vi "FileExplorer.vi"(0 "FolderPath":path, 1 "Copy Button":bool, 2 "Expand/Collapse":bool, 5 "Tree":string[](tree), 7 "SearchBar":string, 11 "error in (no error)":errorcluster) -> (4 "Report":string, 15 "error out":errorcluster)   [LabVIEW 2021]
doc: "This Vi acts as a file explorer. It populates the subfolders and files present in the selected folder path in tree along with the data of Last Modified,Type and Size of files."
uses:
  Controls/Operations.ctl
  Controls/Data Cluster.ctl
  Controls/State.ctl
panel:
  # "Instructions:\n\n-> Select the folder path to populate the subfolders and files present in tree.\n-> A report is generated for the folders whose checkbox is selected in tree.\n-> Press Collapse All button to collapse all nodes in tree and Expand All to expand\n      all nodes in tree.\n->  Enter a folder name in search bar and click enter to expand the nodes of searched folder.\n-> Click column headers such as Last Modified to sort the column itemns in ascending \n      and descending order.\n-> Select file to copy and click Copy button which opens a dialog box to choose the\n      folder path where the files are copied."
  # "Instructions:\n\n-> Select the Folder Path to populate the subfolders and files present in it in tree.\n->  Can select multiple files of same folder and press Copy button to copy those files.\n->  Clicking a Copy button opens a dialog box to choose the destination folder path \n       where the files are copied.\n->  A report is generated for the folders whose checkbox is selected in tree.\n->  Press Collapse All button to collapse all nodes in tree and Expand all to expand \n       all nodes in tree.\n->   Enter a folder name in SearchBar and press Search to search for a particular folder\n       in tree.\n->   Press column headers such as Last Modified to sort the column items in ascending \n        or descending order."
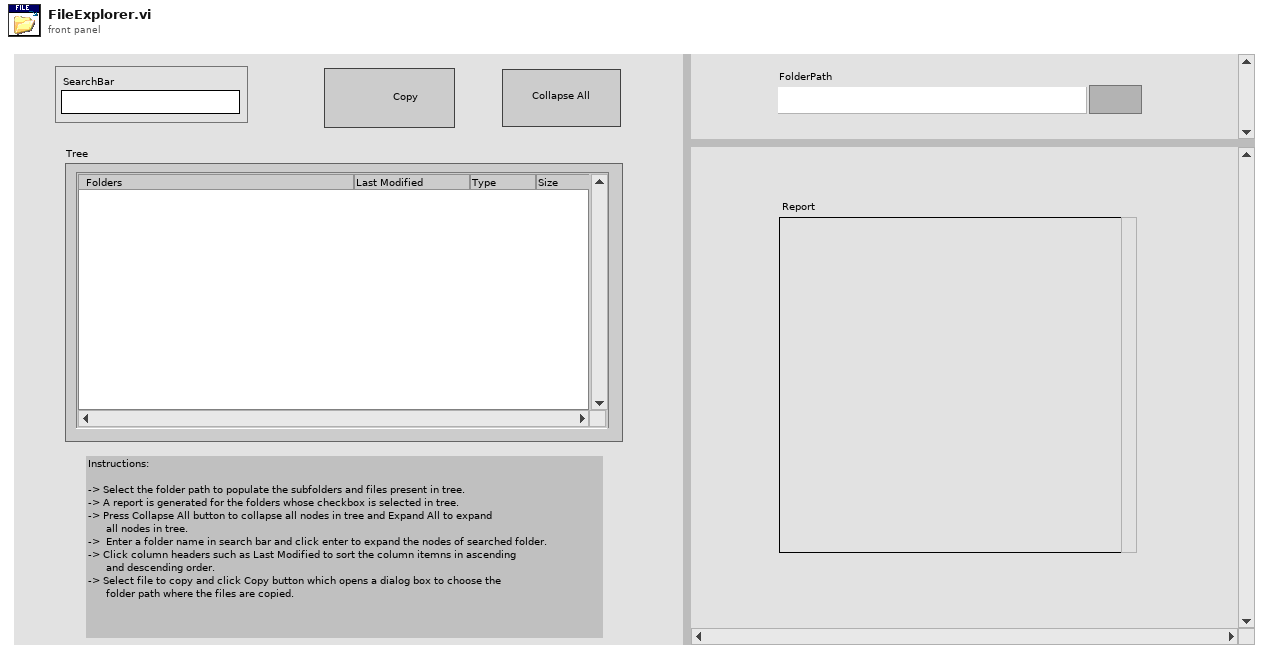
[diagram p1: front panel]
types:
  T1 = typedef "State.ctl" = cluster{"State":string, "Data":variant}
  T2 = typedef "Data Cluster.ctl" = cluster{"Stop user event":refnum<user-event>, "FolderPath":path, "FolderName":string, "FolderPathArray":path[], "FilePathArray":path[], "Index":i32, "No.of Folders":i32, "SelectedTags":string[], "SelectedFilePaths":path[], "SearchTag":string, "Column":i32, "Toggle":bool, "FolderTag":string, "ActiveTag":string, "ListBox":i32, "Report":string, "ValidPath":path, "NewSelectedPath":path}
  T3 = typedef "Operations.ctl" = enum16{"Create", "Enqueue", "Enqueue N", "Enstack", "Dequeue", "Flush", "Release"}
  T4 = typedef "LVPoint32TypeDef.ctl" = cluster{"Horizontal":i32, "Vertical":i32}
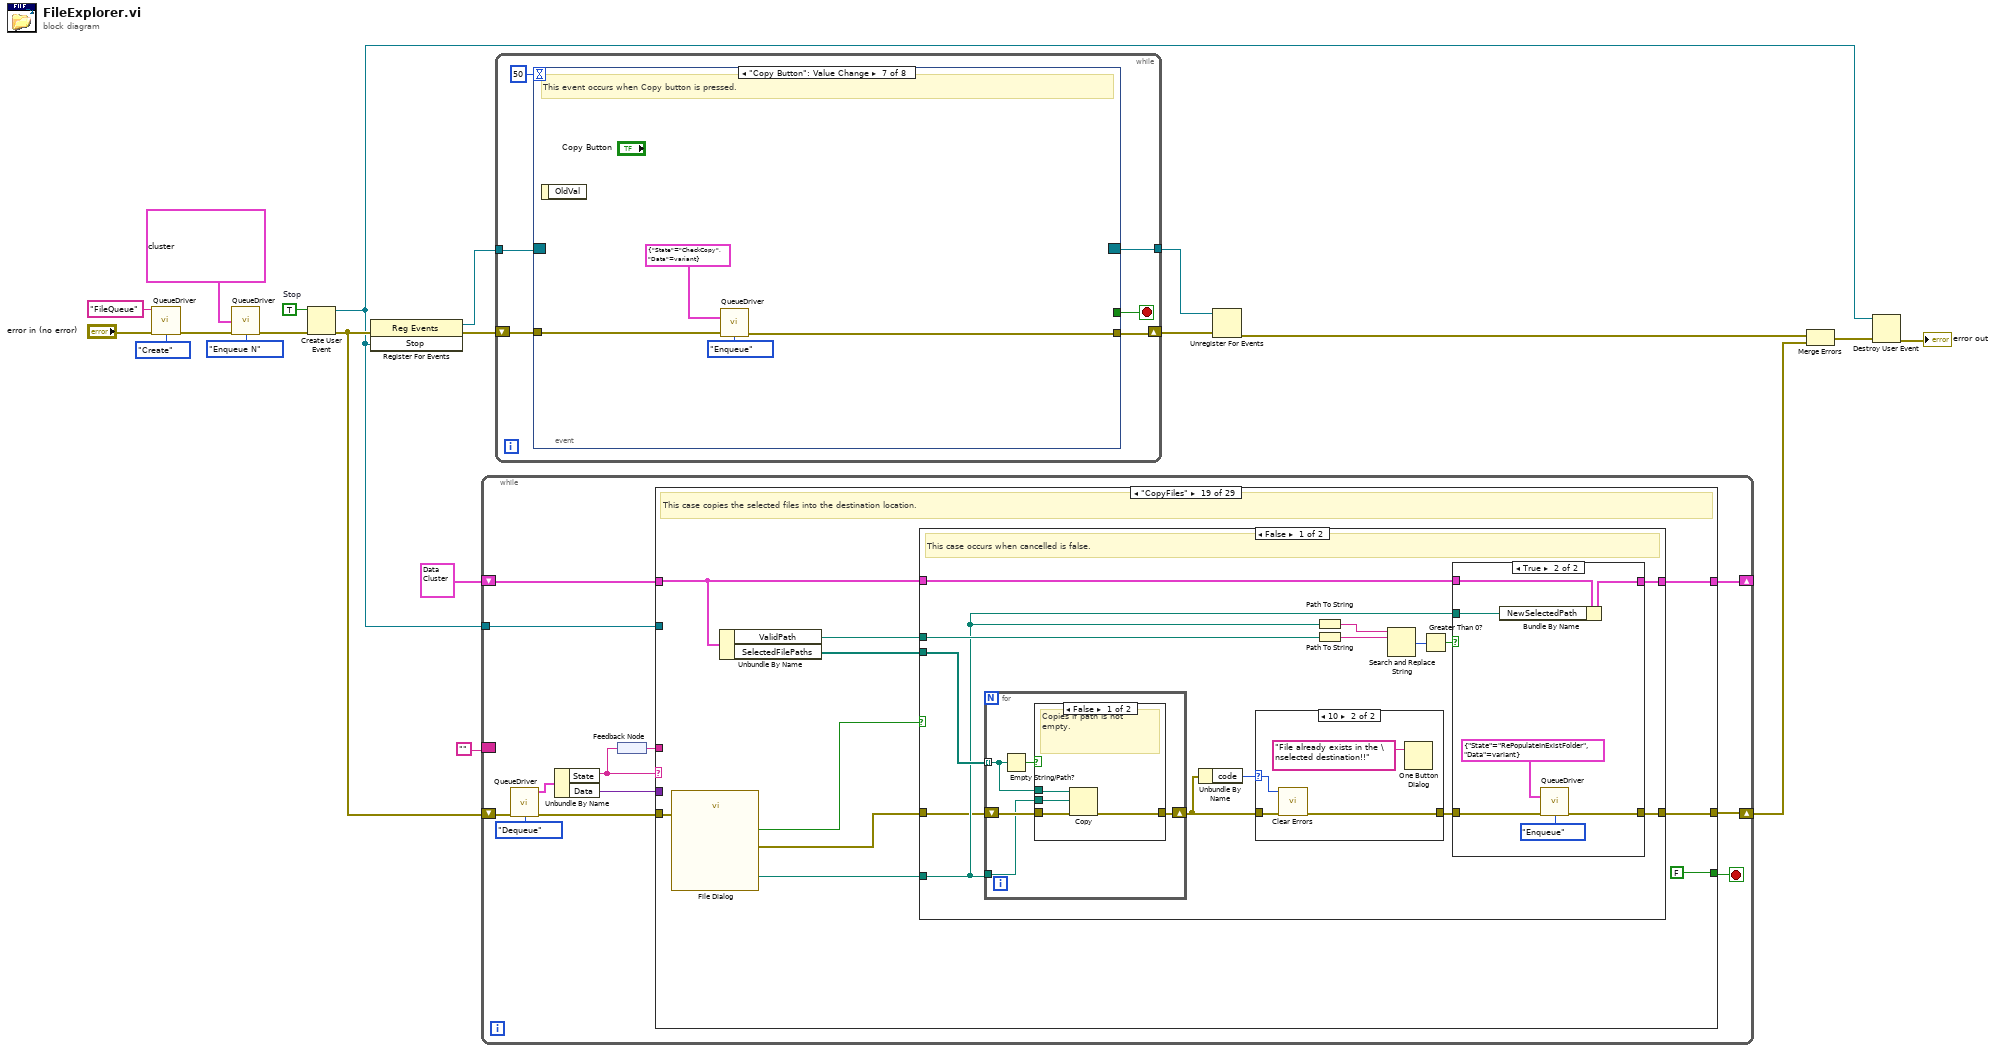
[diagram p0: block diagram]
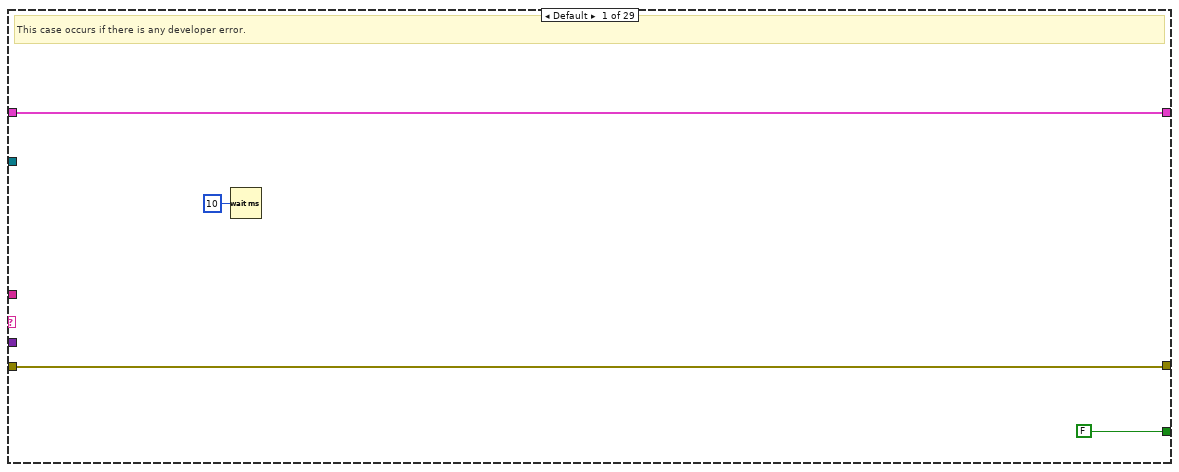
[diagram p2: hidden frame]
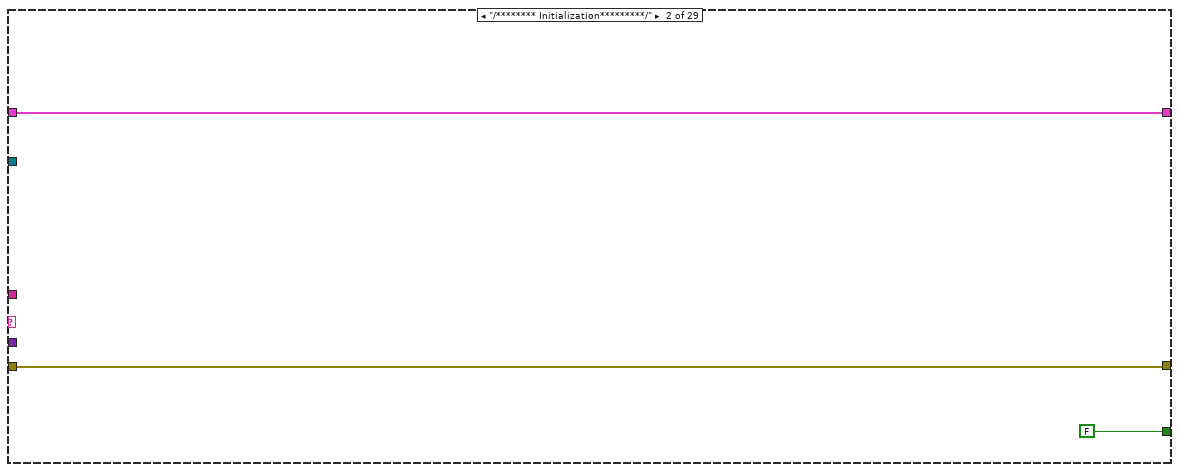
[diagram p3: hidden frame]
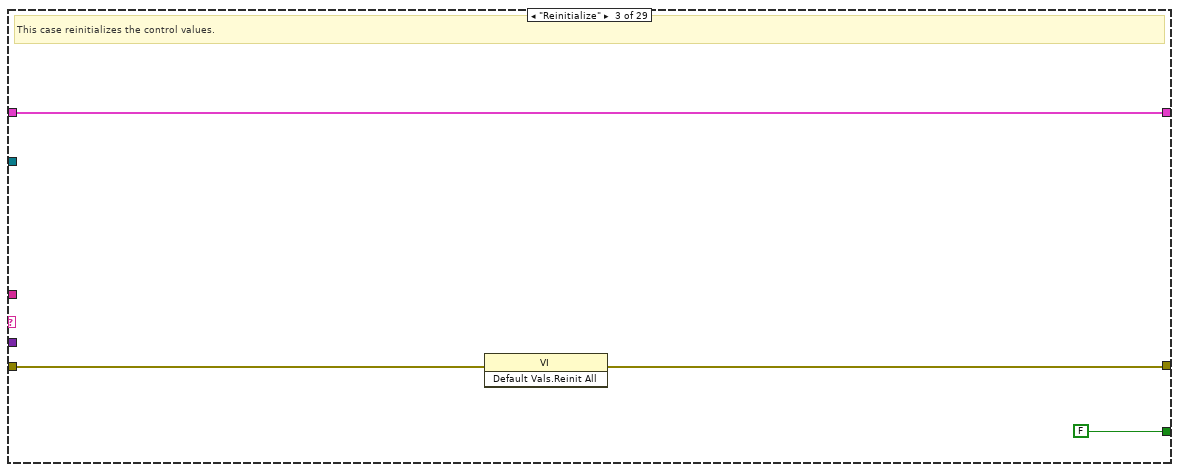
[diagram p4: hidden frame]
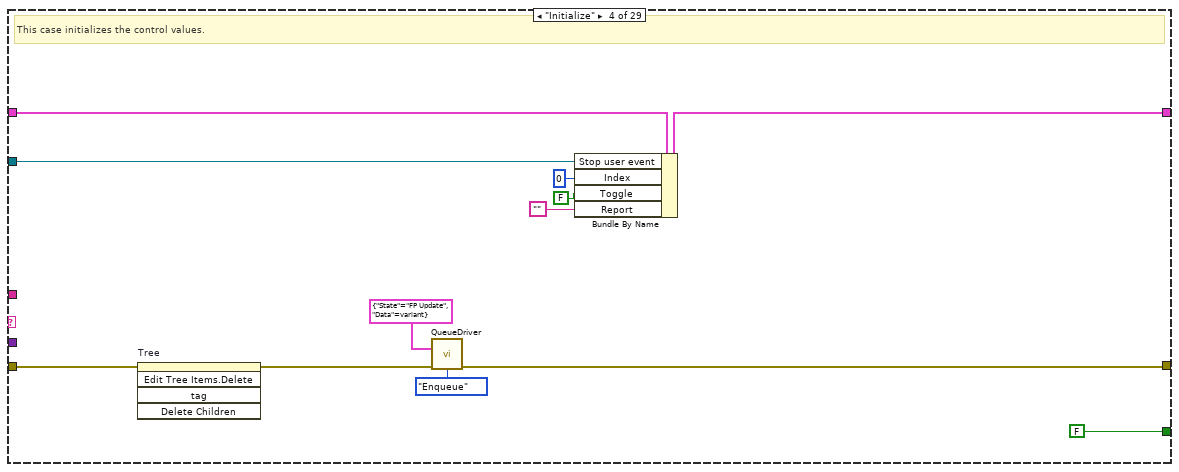
[diagram p5: hidden frame]
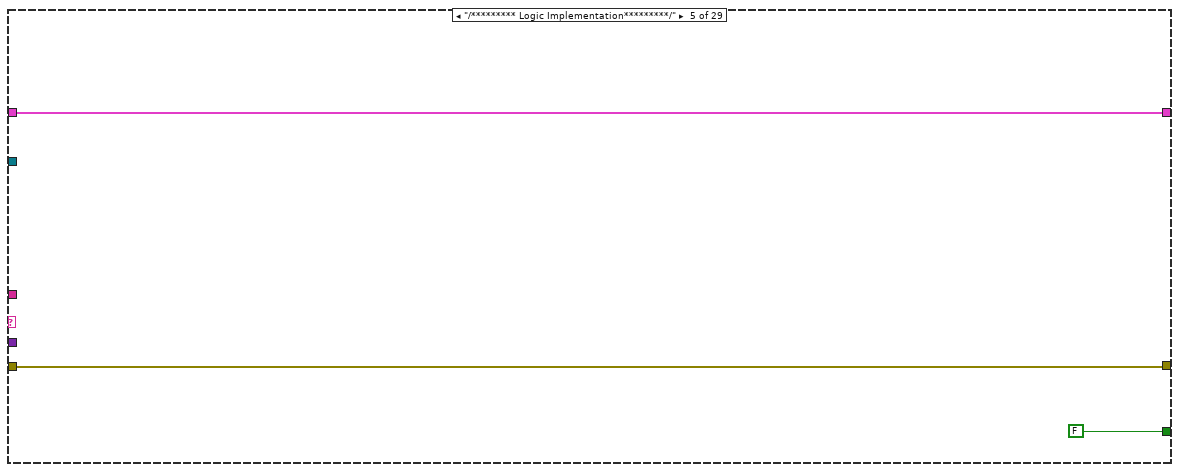
[diagram p6: hidden frame]
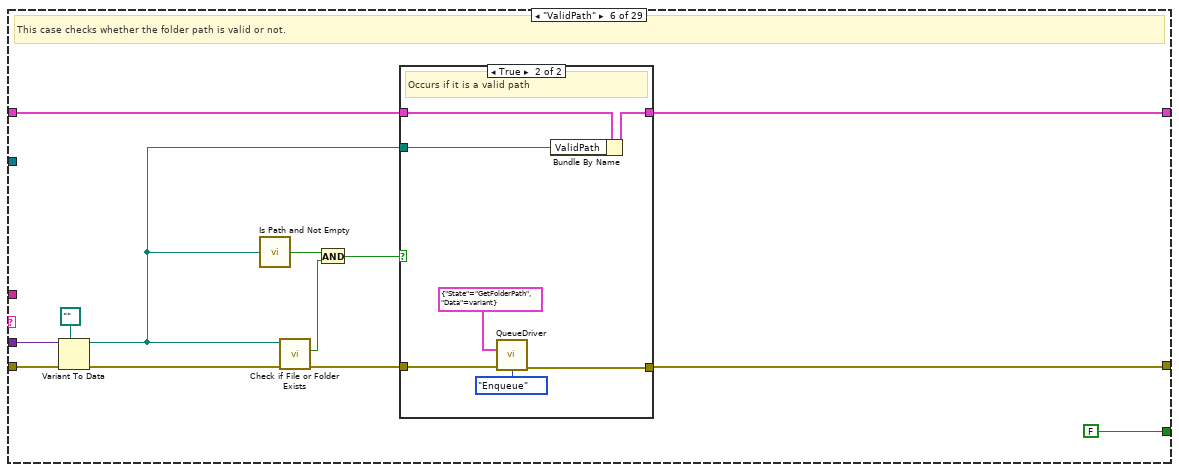
[diagram p7: hidden frame]
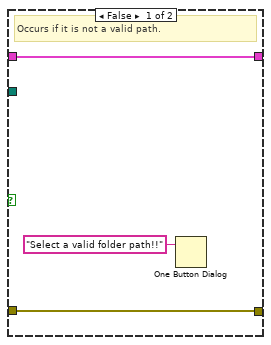
[diagram p8: hidden frame]
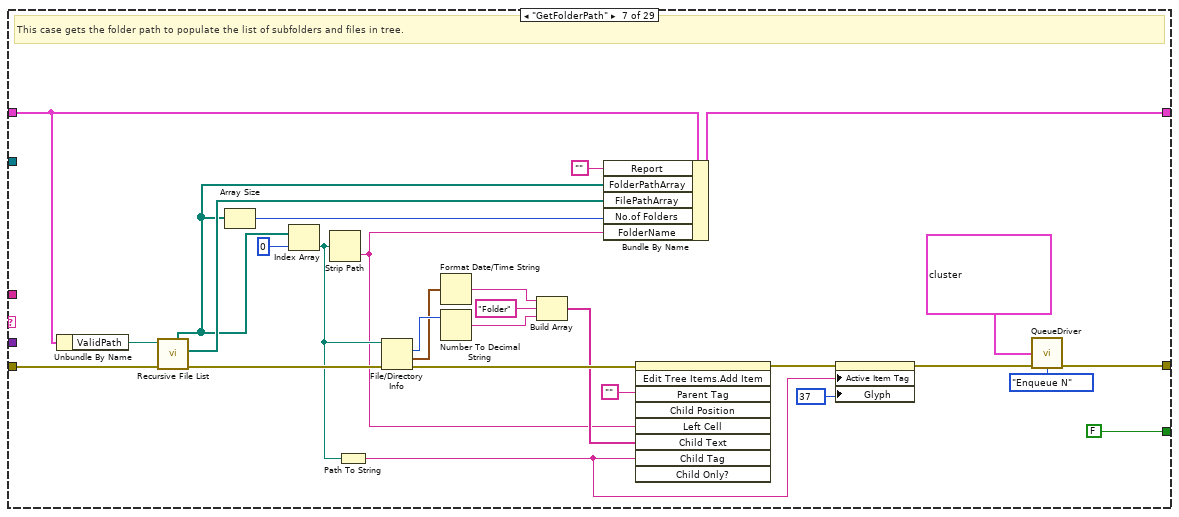
[diagram p9: hidden frame]
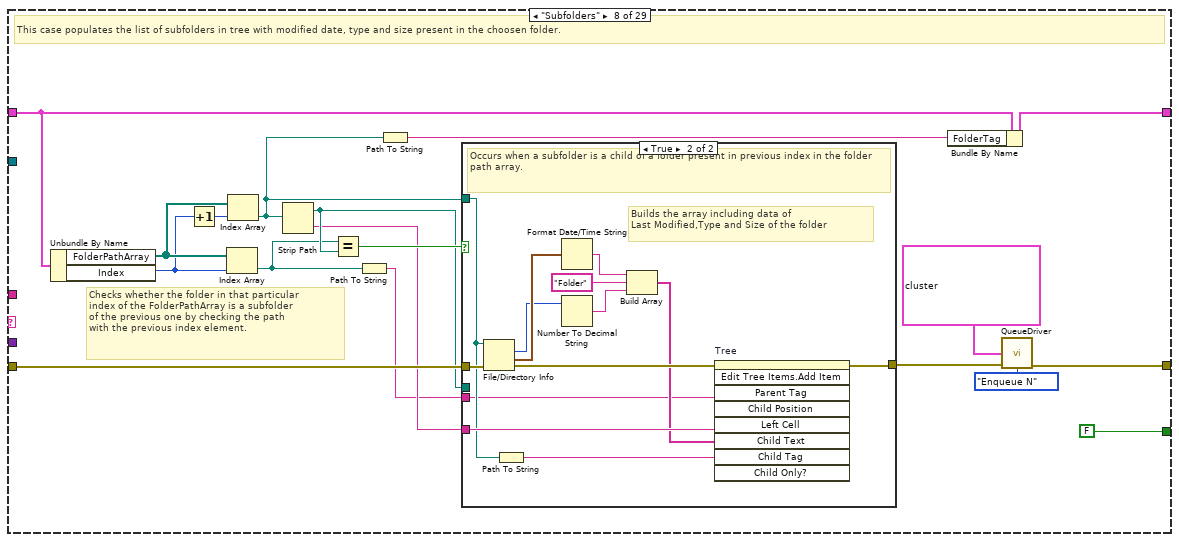
[diagram p10: hidden frame]
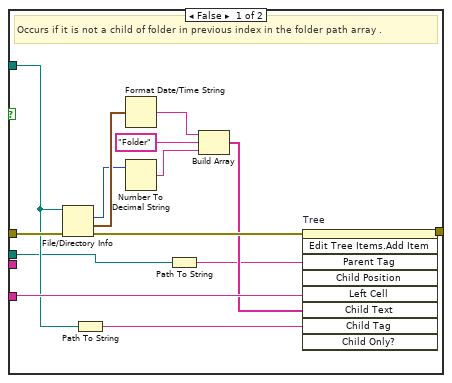
[diagram p11: hidden frame]
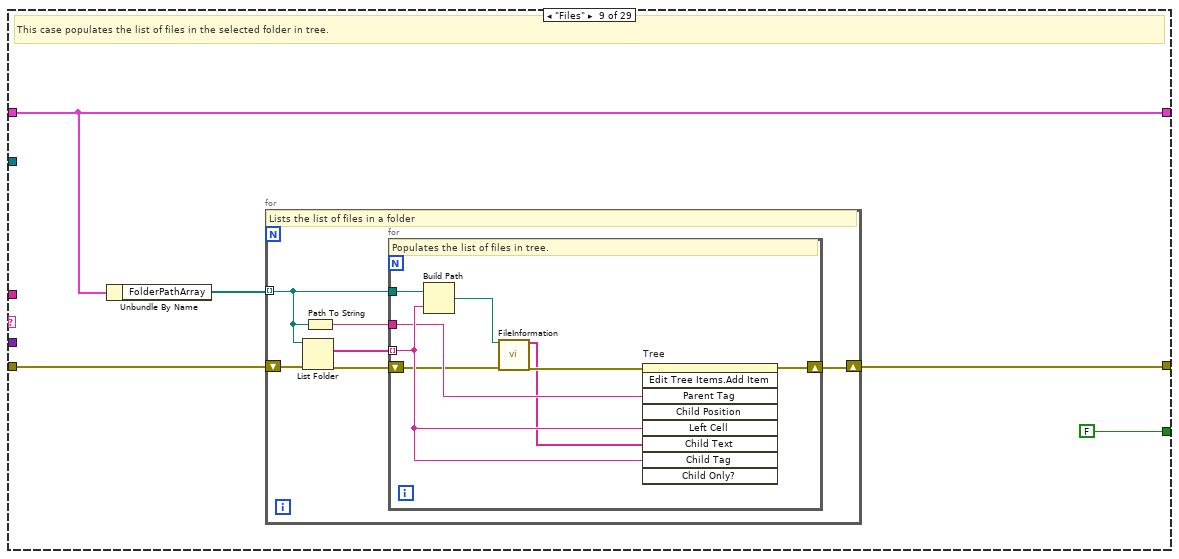
[diagram p12: hidden frame]
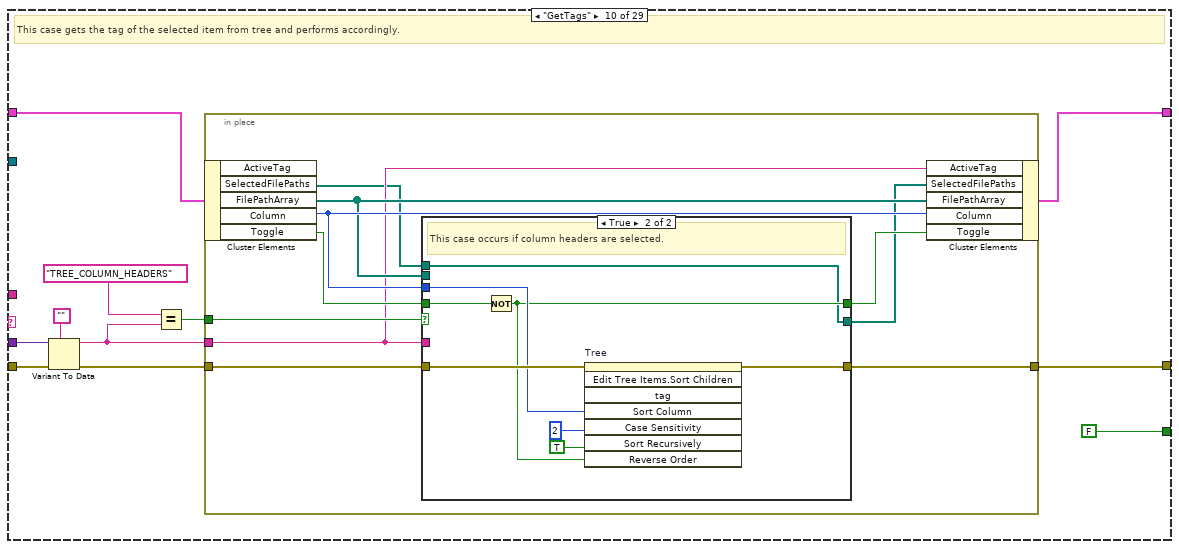
[diagram p13: hidden frame]
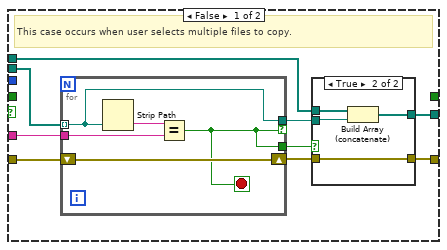
[diagram p14: hidden frame]
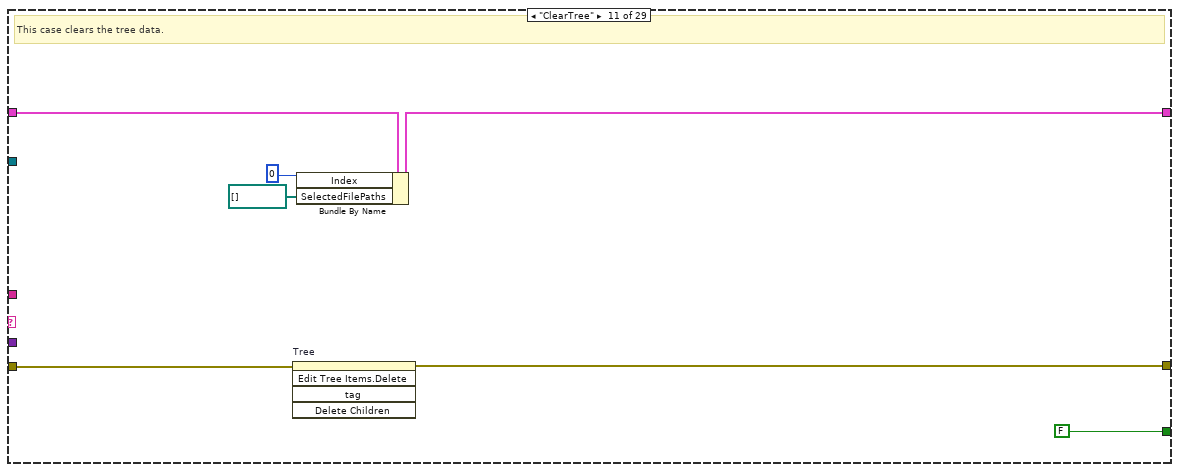
[diagram p16: hidden frame]
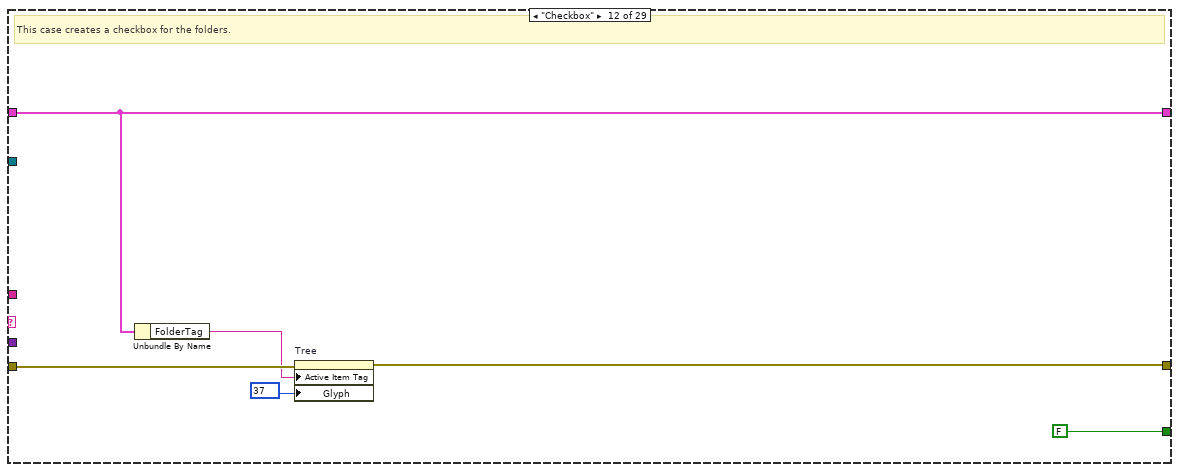
[diagram p17: hidden frame]
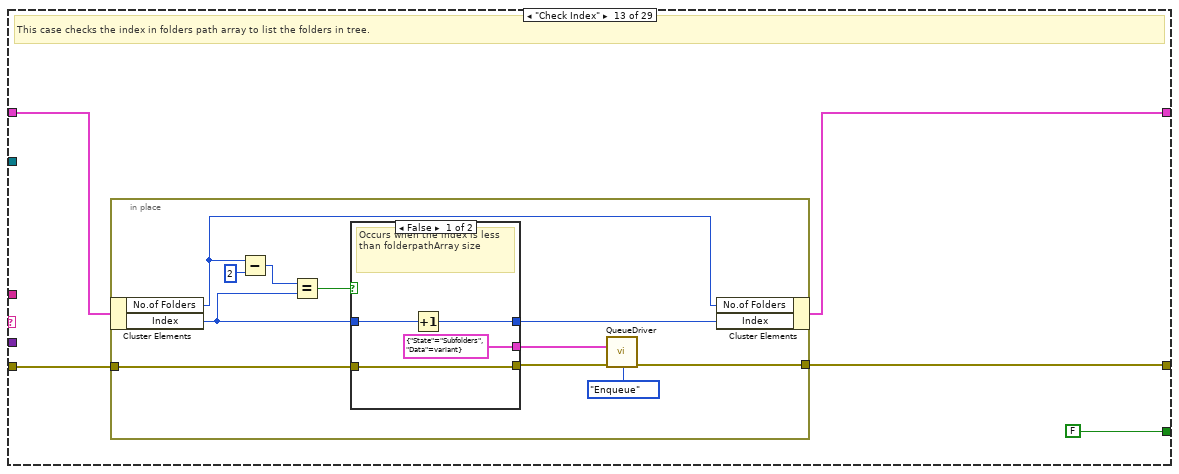
[diagram p18: hidden frame]
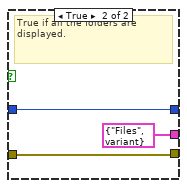
[diagram p19: hidden frame]
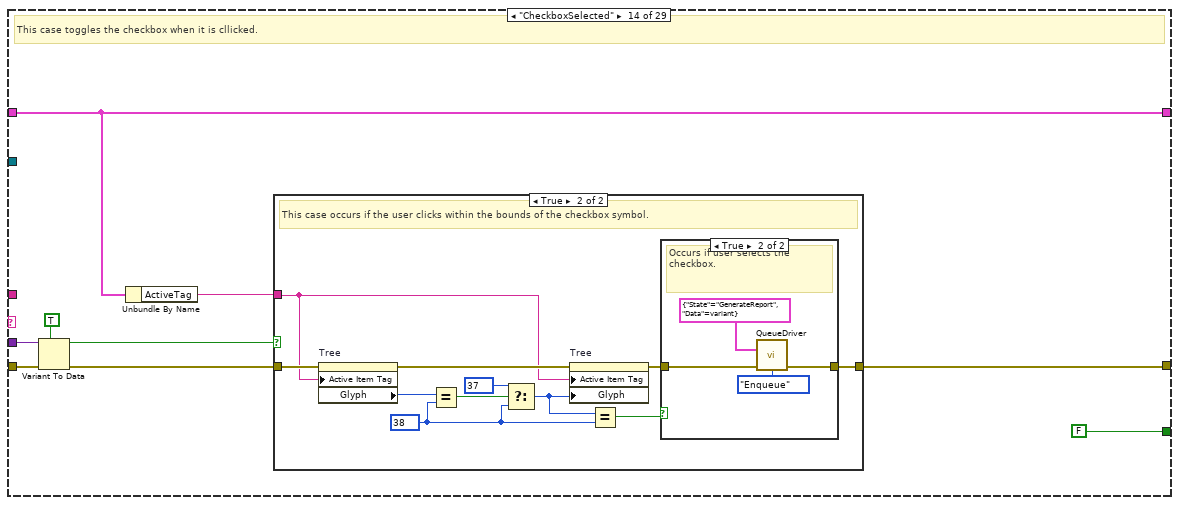
[diagram p20: hidden frame]
diagram:
  w20 = TRUE  # Stop
  n1 = call "QueueDriver.vi"("Queue Name"="FileQueue", "error in (no error)"="error in (no error)", "Operations"=Operations."Create") -> ("error out"=w15:errorcluster)  [unwired: 11 in, 1 out]
  n2 = call "QueueDriver.vi"("State[]"=T1[] [{"State"="Reinitialize", "Data"=variant}, {"State"="Initialize", "Data"=variant}], "error in (no error)"=w15, "Operations"=Operations."Enqueue N") -> ("error out"=w14:errorcluster)  [unwired: 11 in, 1 out]
  n3 = Create User Event(user event datatype=w20, error in=w14) -> (user event=w4:refnum<user-event>, error out=w17:errorcluster)
  n4 = register-events(error in=w17, w4) -> (reference out=w18:refnum<event-registration>, error out=w19:errorcluster)  [unwired: 1 in]
  n5 = while {
    shift-right: [w29] -> w6
    shift-left: w17 -> [w27]
    border: "" ("Empty String Constant") -> [_]
    tunnel: w4 -> [w23]
    shift-right: [w21] -> _
    shift-left: T2 {"Stop user event"=refnum, "FolderPath"=path "", "FolderName"="", "FolderPathArray"=[], "FilePathArray"=[], "Index"=0, "No.of Folders"=0, "SelectedTags"=[], "SelectedFilePaths"=[], "SearchTag"="", "Column"=0, "Toggle"=FALSE, "FolderTag"="", "ActiveTag"="", "ListBox"=0, "Report"="", "ValidPath"=path "", "NewSelectedPath"=path ""} -> [w22]
    stop <- w28 stop-if-true
    n6 = call "QueueDriver.vi"("error in (no error)"=w27, "Operations"=Operations."Dequeue") -> ("Dequeued Element"=w25:T1, "error out"=w26:errorcluster)  [unwired: 12 in]
    n7 = Unbundle By Name(w25) -> ("State"=w32:string, "Data"=w30:variant)
    n8 = feedback-in #1(w32) -> ()
    n9 = feedback #1() -> (w31:string)
    n10 = case shown="\"CopyFiles\"" w32 {
      tunnel: w26 -> [w36 w39 w43 w52 w58 w71 w109 w124 w158 w184 w228 w234 w240 w267 w307 w323 w332 w356 w373 w428 w466 w501 w509 w512 w516 w519 w525 w545 w550]
      tunnel: w31 -> [_ _ _ _ _ _ _ _ _ _ _ _ _ _ _ _ _ _ _ _ _ _ _ _ _ _ w524 _ _]
      tunnel: w30 -> [_ _ _ _ _ w70 _ _ _ w183 _ _ _ w266 _ w322 _ _ _ _ _ w499 w507 _ _ _ _ _ _]
      tunnel: [w36 w39 w41 w46 w58 w68 w105 w120 w156 w181 w229 w233 w239 w260 w288 w317 w324 w355 w370 w423 w464 w496 w508 w512 w516 w519 w523 w545 w549] -> w29
      tunnel: [FALSE FALSE FALSE FALSE FALSE FALSE FALSE FALSE FALSE FALSE FALSE FALSE FALSE FALSE FALSE FALSE FALSE FALSE FALSE FALSE FALSE FALSE FALSE FALSE FALSE FALSE FALSE FALSE TRUE] -> w28
      tunnel: w23 -> [_ _ _ w54 _ _ _ _ _ _ _ _ _ _ _ _ _ _ _ _ _ _ _ _ _ _ _ _ _]
      tunnel: w22 -> [w35 w38 w42 w55 w57 w66 w83 w117 w159 w176 w227 w235 w237 w264 w292 w320 w335 w358 w369 w420 w460 w500 w505 w511 w515 w518 w522 w544 w546]
      tunnel: [w35 w38 w42 w53 w57 w65 w108 w116 w159 w175 w226 w235 w236 w264 w291 w319 w335 w358 w368 w419 w459 w500 w503 w511 w515 w518 w522 w544 w546] -> w21
      frame Default {
        # "This case occurs if there is any developer error."
        n11 = Wait (ms)(milliseconds to wait=u32 10) -> ()  [unwired: 1 out]
      }
      frame "/******** Initialization*********/" {
      }
      frame "Reinitialize" {
        # "This case reinitializes the control values."
        n12 = invoke on="Invoke Node" class="VI" method="Default Vals.Reinit All"(error in=w43) -> (error out=w41:errorcluster)  [unwired: 2 in, 2 out]
      }
      frame "Initialize" {
        # "This case initializes the control values."
        n13 = invoke on="Tree" class="Tree (strict)" method="Edit Tree Items.Delete"(error in=w52) -> (error out=w49:errorcluster)  [unwired: 4 in, 4 out]
        n14 = call "QueueDriver.vi"("State"=T1 {"State"="FP Update", "Data"=variant}, "error in (no error)"=w49, "Operations"=Operations."Enqueue") -> ("error out"=w46:errorcluster)  [unwired: 11 in, 1 out]
        n15 = Bundle By Name(cluster=w55, "Stop user event"=w54, "Index"=0, "Toggle"=FALSE, "Report"="" ("Empty String Constant")) -> (w53:T2)
      }
      frame "/********* Logic Implementation*********/" {
      }
      frame "ValidPath" {
        # "This case checks whether the folder path is valid or not."
        n16 = Variant To Data(error in=w71, type=path "", Variant=w70) -> (data=w61:path, error out=w64:errorcluster)
        n17 = call <vilib>:"Is Path and Not Empty.vi"("path"=w61) -> ("Is Path and Not Empty?"=w60:bool)  [unwired: 4 in]
        n18 = call <vilib>:"Check if File or Folder Exists.vi"("error in (no error)"=w64, "path"=w61) -> ("error out"=w63:errorcluster, "file or folder exists?"=w62:bool)  [unwired: 7 in, 1 out]
        n19 = And(x=w60, y=w62) -> (x .and. y?=w59:bool)
        n20 = case shown="True" w59 {
          tunnel: w63 -> [w74 w81]
          tunnel: [w74 w80] -> w68
          tunnel: w66 -> [w72 w77]
          tunnel: w61 -> [_ w76]
          tunnel: [w72 w75] -> w65
          frame False {
            # "Occurs if it is not a valid path."
            n21 = One Button Dialog(message="Select a valid folder path!!") -> ()  [unwired: 1 in, 1 out]
          }
          frame True {
            # "Occurs if it is a valid path"
            n22 = call "QueueDriver.vi"("State"=T1 {"State"="GetFolderPath", "Data"=variant}, "error in (no error)"=w81, "Operations"=Operations."Enqueue") -> ("error out"=w80:errorcluster)  [unwired: 11 in, 1 out]
            n23 = Bundle By Name(cluster=w77, "ValidPath"=w76) -> (w75:T2)
          }
        }
      }
      frame "GetFolderPath" {
        # "This case gets the folder path to populate the list of subfolders and files in tree."
        n24 = Unbundle By Name(w83) -> ("ValidPath"=w82:path)
        n25 = call <vilib>:"Recursive File List.vi"("error in (no error)"=w109, "Folder Path"=w82) -> ("error out"=w98:errorcluster, "All Files in Dir"=w107:path[], "All Folders"=w103:path[])  [unwired: 5 in, 2 out]
        n26 = Array Size(array=w103) -> (size(s)=w102:i32)
        n27 = Index Array(array=w103, index=0) -> (element=w86:path)
        n28 = Strip Path(path=w86) -> (name=w85:string)  [unwired: 1 out]
        n29 = Path To String(path=w86) -> (string=w84:string)
        n30 = File/Directory Info(path=w86, error in=w98) -> (size=w99:i64, last mod=w96:timestamp, error out=w97:errorcluster)  [unwired: 4 out]
        n31 = Format Date/Time String(seconds (now)=w96) -> (date/time string=w95:string)  [unwired: 2 in]
        n32 = Number To Decimal String(number=w99) -> (decimal integer string=w100:string)  [unwired: 1 in]
        n33 = Build Array(w95, "Folder" ("element"), w100) -> (w94:string[])
        n34 = Bundle By Name(cluster=w83, "Report"="" ("Empty String Constant"), "FolderPathArray"=w103, "FilePathArray"=w107, "No.of Folders"=w102, "FolderName"=w85) -> (w108:T2)
        n35 = invoke on="Tree" class="Tree (strict)" method="Edit Tree Items.Add Item"(error in=w97, "Parent Tag"="" ("Empty String Constant"), "Left Cell"=w85, "Child Text"=w94, "Child Tag"=w84) -> (error out=w93:errorcluster)  [unwired: 4 in, 8 out]
        n36 = property on="Tree" class="Tree (strict)"(error in=w93, "Active Item Tag"=w84, "Glyph"=37) -> (error out=w92:errorcluster)  [unwired: 1 in, 1 out]
        n37 = call "QueueDriver.vi"("State[]"=T1[] [{"State"="FP Update", "Data"=variant}, {"State"="Subfolders", "Data"=variant}], "error in (no error)"=w92, "Operations"=Operations."Enqueue N") -> ("error out"=w105:errorcluster)  [unwired: 11 in, 1 out]
      }
      frame "Subfolders" {
        # "Checks whether the folder in that particular\nindex of the FolderPathArray is a subfolder \nof the previous one by checking the path\nwith the previous index element."
        # "This case populates the list of subfolders in tree with modified date, type and size present in the choosen folder."
        n38 = Unbundle By Name(w117) -> ("FolderPathArray"=w127:path[], "Index"=w126:i32)
        n39 = Increment(x=w126) -> (x+1=w125:i32)
        n40 = Index Array(array=w127, index=w126) -> (element=w111:path)
        n41 = Index Array(array=w127, index=w125) -> (element=w113:path)
        n42 = Strip Path(path=w113) -> (stripped path=w122:path, name=w115:string)
        n43 = Equal?(x=w111, y=w122) -> (x = y?=w123:bool)
        n44 = Path To String(path=w111) -> (string=w110:string)
        n45 = Path To String(path=w113) -> (string=w112:string)
        n46 = case shown="True" w123 {
          tunnel: w124 -> [w136 w150]
          tunnel: [w141 w154] -> w121
          tunnel: w115 -> [w140 w153]
          tunnel: w122 -> [w129 _]
          tunnel: w113 -> [w131 w144]
          tunnel: w110 -> [_ w142]
          frame False {
            # "Occurs if it is not a child of folder in previous index in the folder path array ."
            n47 = File/Directory Info(path=w131, error in=w136) -> (size=w133:i64, last mod=w134:timestamp, error out=w135:errorcluster)  [unwired: 4 out]
            n48 = Path To String(path=w131) -> (string=w130:string)
            n49 = Format Date/Time String(seconds (now)=w134) -> (date/time string=w139:string)  [unwired: 2 in]
            n50 = Number To Decimal String(number=w133) -> (decimal integer string=w137:string)  [unwired: 1 in]
            n51 = Path To String(path=w129) -> (string=w128:string)
            n52 = Build Array(w139, "Folder" ("element"), w137) -> (w132:string[])
            n53 = invoke on="Tree" class="Tree (strict)" method="Edit Tree Items.Add Item"(error in=w135, "Parent Tag"=w128, "Left Cell"=w140, "Child Text"=w132, "Child Tag"=w130) -> (error out=w141:errorcluster)  [unwired: 4 in, 8 out]
          }
          frame True {
            # "Builds the array including data of\nLast Modified,Type and Size of the folder"
            # "Occurs when a subfolder is a child of a folder present in previous index in the folder path array."
            n54 = File/Directory Info(path=w144, error in=w150) -> (size=w151:i64, last mod=w152:timestamp, error out=w149:errorcluster)  [unwired: 4 out]
            n55 = Path To String(path=w144) -> (string=w143:string)
            n56 = Format Date/Time String(seconds (now)=w152) -> (date/time string=w148:string)  [unwired: 2 in]
            n57 = Number To Decimal String(number=w151) -> (decimal integer string=w146:string)  [unwired: 1 in]
            n58 = Build Array(w148, "Folder" ("element"), w146) -> (w145:string[])
            n59 = invoke on="Tree" class="Tree (strict)" method="Edit Tree Items.Add Item"(error in=w149, "Parent Tag"=w142, "Left Cell"=w153, "Child Text"=w145, "Child Tag"=w143) -> (error out=w154:errorcluster)  [unwired: 4 in, 8 out]
          }
        }
        n60 = Bundle By Name(cluster=w117, "FolderTag"=w112) -> (w116:T2)
        n61 = call "QueueDriver.vi"("State[]"=T1[] [{"State"="Checkbox", "Data"=variant}, {"State"="Check Index", "Data"=variant}], "error in (no error)"=w121, "Operations"=Operations."Enqueue N") -> ("error out"=w120:errorcluster)  [unwired: 11 in, 1 out]
      }
      frame "Files" {
        # "This case populates the list of files in the selected folder in tree."
        n62 = Unbundle By Name(w159) -> ("FolderPathArray"=w157:path[])
        n63 = for {
          shift-right: [w165] -> w156
          shift-left: w158 -> [w163]
          tunnel: w157 -> [w160] mode=indexing
          # "Lists the list of files in a folder"
          n64 = List Folder(path=w160, error in=w163) -> (filenames=w161:string[], error out=w162:errorcluster)  [unwired: 2 in, 2 out]
          n65 = Path To String(path=w160) -> (string=w164:string)
          n66 = for {
            shift-right: [w173] -> w165
            shift-left: w162 -> [w169]
            tunnel: w164 -> [w170]
            tunnel: w161 -> [w171] mode=indexing
            tunnel: w160 -> [w172]
            # "Populates the list of files in tree."
            n67 = Build Path(base path=w172, name or relative path=w171) -> (appended path=w167:path)
            n68 = call "FileInformation.vi"("File Path"=w167, "error in (no error)"=w169) -> ("FileInfo"=w166:string[], "error out"=w168:errorcluster)  [unwired: 12 in]
            n69 = invoke on="Tree" class="Tree (strict)" method="Edit Tree Items.Add Item"(error in=w168, "Parent Tag"=w170, "Left Cell"=w171, "Child Text"=w166, "Child Tag"=w171) -> (error out=w173:errorcluster)  [unwired: 4 in, 8 out]
          }
        }
      }
      frame "GetTags" {
        # "This case gets the tag of the selected item from tree and performs accordingly."
        n70 = Variant To Data(error in=w184, type="" ("Empty String Constant"), Variant=w183) -> (data=w178:string, error out=w182:errorcluster)
        n71 = Equal?(x="TREE_COLUMN_HEADERS", y=w178) -> (x = y?=w179:bool)
        n72 = in-place "In Place Element Structure" {
          in-place-border: w182 -> [w194]
          in-place-border: [w193] -> w181
          in-place-border: w179 -> [w192]
          in-place-border: w178 -> [w187]
          n73 = in-place-cluster #2(w176) -> ("SelectedFilePaths"=w186:path[], "FilePathArray"=w188:path[], "Column"=w189:i32, "Toggle"=w191:bool)  [unwired: 1 out]
          n74 = case shown="True" w192 {
            tunnel: w194 -> [w201 w222]
            tunnel: w188 -> [w203 _]
            tunnel: [w196 w221] -> w193
            tunnel: w187 -> [w202 _]
            tunnel: w189 -> [_ w220]
            tunnel: w191 -> [_ w217]
            tunnel: [_ w216] -> w190
            tunnel: w186 -> [w199 w215]
            tunnel: [w197 w215] -> w185
            frame False {
              # "This case occurs when user selects multiple files to copy."
              n75 = for {
                tunnel: w203 -> [w211] mode=indexing
                tunnel: w202 -> [w213]
                tunnel: [w211] -> w198 if=w210
                shift-right: [w212] -> w195
                shift-left: w201 -> [w212]
                tunnel: [w210] -> w200
                stop <- w210 stop-if-true
                n76 = Strip Path(path=w211) -> (name=w214:string)  [unwired: 1 out]
                n77 = Equal?(x=w214, y=w213) -> (x = y?=w210:bool)
              }
              n78 = case shown="True" w200 {
                tunnel: w199 -> [w204 w209]
                tunnel: w198 -> [_ w208]
                tunnel: [w204 w207] -> w197
                tunnel: [w205 w206] -> w196
                tunnel: w195 -> [w205 w206]
                frame False {
                }
                frame True {
                  n79 = Build Array (concatenate)(w209, w208) -> (w207:path[])
                }
              }
            }
            frame True {
              # "This case occurs if column headers are selected."
              n80 = Not(x=w217) -> (.not. x?=w216:bool)
              n81 = invoke on="Tree" class="Tree (strict)" method="Edit Tree Items.Sort Children"(error in=w222, "Sort Column"=w220, "Case Sensitivity"=2, "Sort Recursively"=TRUE ("Sort Recursively?"), "Reverse Order"=w216) -> (error out=w221:errorcluster)  [unwired: 3 in, 7 out]
            }
          }
          n82 = in-place-cluster #2("ActiveTag"=w187, "SelectedFilePaths"=w185, "FilePathArray"=w188, "Column"=w189, "Toggle"=w190) -> (w175:T2)
        }
      }
      frame "ClearTree" {
        # "This case clears the tree data."
        n83 = invoke on="Tree" class="Tree (strict)" method="Edit Tree Items.Delete"(error in=w228) -> (error out=w229:errorcluster)  [unwired: 4 in, 4 out]
        n84 = Bundle By Name(cluster=w227, "Index"=0, "SelectedFilePaths"=path[] []) -> (w226:T2)
      }
      frame "Checkbox" {
        # "This case creates a checkbox for the folders."
        n85 = Unbundle By Name(w235) -> ("FolderTag"=w232:string)
        n86 = property on="Tree" class="Tree (strict)"(error in=w234, "Active Item Tag"=w232, "Glyph"=37) -> (error out=w233:errorcluster)  [unwired: 1 in, 1 out]
      }
      frame "Check Index" {
        # "This case checks the index in folders path array to list the folders in tree."
        n87 = in-place "In Place Element Structure" {
          in-place-border: w240 -> [w249]
          in-place-border: [w244] -> w239
          n88 = in-place-cluster #3(w237) -> ("No.of Folders"=w241:i32, "Index"=w243:i32)
          n89 = Subtract(x=w241, y=2) -> (x-y=w250:i32)
          n90 = Equal?(x=w250, y=w243) -> (x = y?=w248:bool)
          n91 = case shown="False" w248 {
            tunnel: w249 -> [w254 w258]
            tunnel: [w254 w258] -> w247
            tunnel: [T1 {"State"="Subfolders", "Data"=variant} ("State") T1 {"State"="Files", "Data"=variant} ("State")] -> w245
            tunnel: w243 -> [w253 w256]
            tunnel: [w252 w256] -> w242
            frame False {
              # "Occurs when the index is less than folderpathArray size"
              n92 = Increment(x=w253) -> (x+1=w252:i32)
            }
            frame True {
              # "True if all the folders are displayed."
            }
          }
          n93 = call "QueueDriver.vi"("State"=w245, "error in (no error)"=w247, "Operations"=Operations."Enqueue") -> ("error out"=w244:errorcluster)  [unwired: 11 in, 1 out]
          n94 = in-place-cluster #3("No.of Folders"=w241, "Index"=w242) -> (w236:T2)
        }
      }
      frame "CheckboxSelected" {
        # "This case toggles the checkbox when it is cllicked."
        n95 = Variant To Data(error in=w267, type=TRUE, Variant=w266) -> (data=w263:bool, error out=w261:errorcluster)
        n96 = Unbundle By Name(w264) -> ("ActiveTag"=w262:string)
        n97 = case shown="True" w263 {
          tunnel: w262 -> [_ w274]
          tunnel: w261 -> [w268 w279]
          tunnel: [w268 w269] -> w260
          frame False {
            # "This case occurs if it is not within the bounds of the symbol."
          }
          frame True {
            w272 = 38
            # "This case occurs if the user clicks within the bounds of the checkbox symbol."
            n98 = property on="Tree" class="Tree (strict)"(error in=w279, "Active Item Tag"=w274) -> (error out=w275:errorcluster, "Glyph"=w278:i32)  [unwired: 1 in, 1 out]
            n99 = Equal?(x=w278, y=w272) -> (x = y?=w277:bool)
            n100 = Select(t=37, s=w277, f=w272) -> (s? t:f=w273:i32)
            n101 = property on="Tree" class="Tree (strict)"(error in=w275, "Active Item Tag"=w274, "Glyph"=w273) -> (error out=w271:errorcluster)  [unwired: 1 in, 1 out]
            n102 = Equal?(x=w273, y=w272) -> (x = y?=w270:bool)
            n103 = case shown="True" w270 {
              tunnel: w271 -> [w280 w284]
              tunnel: [w280 w283] -> w269
              frame False {
                # "Occurs if it is unchecked."
              }
              frame True {
                # "Occurs if user selects the checkbox."
                n104 = call "QueueDriver.vi"("State"=T1 {"State"="GenerateReport", "Data"=variant}, "error in (no error)"=w284, "Operations"=Operations."Enqueue") -> ("error out"=w283:errorcluster)  [unwired: 11 in, 1 out]
              }
            }
          }
        }
      }
      frame "GenerateReport" {
        # "Generates a report including LastModified, Type and Size of the selected folder."
        n105 = Unbundle By Name(w292) -> ("Report"=w294:string, "FolderPathArray"=w303:path[], "ActiveTag"=w302:string)
        n106 = property on="Tree" class="Tree (strict)"(error in=w307, "Active Item Tag"=w302, "ActiveColNum"=1 ("Active Cell:Active Column Number"), "ActiveColNum"=2 ("Active Cell:Active Column Number"), "ActiveColNum"=3 ("Active Cell:Active Column Number")) -> (error out=w301:errorcluster, "Cell String"=w297:string, "Cell String"=w296:string, "Cell String"=w295:string)  [unwired: 1 in, 1 out]
        n107 = for {
          tunnel: w303 -> [w308] mode=indexing
          tunnel: w302 -> [w314]
          tunnel: [w313] -> w298
          shift-right: [w312] -> w300
          shift-left: w301 -> [w312]
          stop <- w309 stop-if-true
          # "Gets the folder path of selected folder."
          n108 = Strip Path(path=w308) -> (name=w315:string)  [unwired: 1 out]
          n109 = Equal?(x=w315, y=w314) -> (x = y?=w309:bool)
          n110 = Select(t=w308, s=w309, f=path "") -> (s? t:f=w311:path)
          n111 = Path To String(path=w311) -> (string=w313:string)
        }
        n112 = Format Into String(format string="Path: %s\nLast Modified: %s\nType: %s\nSize: %s\n<--------------------------------------------------------->\n", error in=w300, w298, w297, w296, w295) -> (resulting string=w293:string, error out=w289:errorcluster)  [unwired: 1 in]
        n113 = Concatenate Strings(w294, w293) -> (w290:string)
        n114 = Bundle By Name(cluster=w292, "Report"=w290) -> (w291:T2)
        n115 = call "QueueDriver.vi"("State"=T1 {"State"="FP Update", "Data"=variant}, "error in (no error)"=w289, "Operations"=Operations."Enqueue") -> ("error out"=w288:errorcluster)  [unwired: 11 in, 1 out]
      }
      frame "SearchTag" {
        # "This case gets the folder name that user enters in SearchBar."
        n116 = Variant To Data(error in=w323, type="" ("Empty String Constant"), Variant=w322) -> (data=w318:string, error out=w317:errorcluster)
        n117 = Bundle By Name(cluster=w320, "SearchTag"=w318) -> (w319:T2)
      }
      frame "SearchFolder" {
        # "This case expands the contents of the searched folder."
        n118 = Unbundle By Name(w335) -> ("SearchTag"=w330:string, "FolderPathArray"=w331:path[])
        n119 = for {
          tunnel: w331 -> [w344] mode=indexing
          tunnel: w330 -> [w345]
          tunnel: [w344] -> w329 if=w343
          shift-right: [w342] -> w327
          shift-left: w332 -> [w342]
          stop <- w343 stop-if-true
          n120 = Strip Path(path=w344) -> (name=w346:string)  [unwired: 1 out]
          n121 = Equal?(x=w346, y=w345) -> (x = y?=w343:bool)
        }
        n122 = Empty String/Path?(string/path=w330) -> (empty?=w334:bool)
        n123 = Path To String(path=w329) -> (string=w328:string)
        n124 = case shown="False" w334 {
          tunnel: w327 -> [w351 w352]
          tunnel: [w349 w352] -> w325
          tunnel: w328 -> [w347 _]
          frame False {
            # "Occurs if the string is not empty."
            n125 = invoke on="Tree" class="Tree (strict)" method="Open/Close.Ensure Visible"(error in=w351, "tag"=w347) -> (error out=w350:errorcluster)  [unwired: 2 in, 3 out]
            n126 = invoke on="Tree" class="Tree (strict)" method="Open/Close.Item"(error in=w350, "tag"=w347, "Open"=TRUE ("Open?")) -> (error out=w349:errorcluster)  [unwired: 2 in, 4 out]
          }
          frame True {
            # "Occurs if string is empty."
          }
        }
        n127 = Unbundle By Name(w325) -> ("code"=w326:i32)
        n128 = case shown="1" w326 {
          selector: w326 -> [_ w339]
          tunnel: w325 -> [w336 w340]
          tunnel: [w336 w338] -> w324
          frame 0, Default {
          }
          frame 1 {
            n129 = call <vilib>:"Clear Errors.vi"("error in (no error)"=w340, "specific error code to clear (0: all)"=w339) -> ("error out"=w338:errorcluster)  [unwired: 4 in, 1 out]
            n130 = local write "SearchBar"("" ("Empty String Constant")) -> ()
            n131 = One Button Dialog(message="Invalid folder name!!\nEnter a valid folder name\nname to search") -> ()  [unwired: 1 in, 1 out]
          }
        }
      }
      frame "CheckCopy" {
        # "Checks whether the files are selected for copy."
        n132 = Unbundle By Name(w358) -> ("SelectedFilePaths"=w357:path[])
        n133 = Empty Array?(array=w357) -> (empty?=w354:bool)
        n134 = case shown="False" w354 {
          tunnel: w356 -> [w362 w364]
          tunnel: [w361 w364] -> w355
          frame False {
            # "Occurs if files are selected in tree."
            n135 = call "QueueDriver.vi"("State"=T1 {"State"="CopyFiles", "Data"=variant}, "error in (no error)"=w362, "Operations"=Operations."Enqueue") -> ("error out"=w361:errorcluster)  [unwired: 11 in, 1 out]
          }
          frame True {
            # "Occurs if no file is selected."
            n136 = One Button Dialog(message="Files not selected!!\nSelect files to copy") -> ()  [unwired: 1 in, 1 out]
          }
        }
      }
      frame "CopyFiles" {
        # "This case copies the selected files into the destination location."
        n137 = call "File Dialog"("error in"=w373) -> ("selected path"=w367:path, "cancelled"=w365:bool, "error out"=w366:errorcluster)  [unwired: 11 in, 1 out]
        n138 = Unbundle By Name(w369) -> ("ValidPath"=w371:path, "SelectedFilePaths"=w374:path[])
        n139 = case shown="False" w365 {
          tunnel: w374 -> [w388 _]
          tunnel: w371 -> [w387 _]
          tunnel: [w382 w417] -> w370
          tunnel: w369 -> [w381 w415]
          tunnel: [w380 w415] -> w368
          tunnel: w367 -> [w379 _]
          tunnel: w366 -> [w375 w418]
          frame False {
            # "This case occurs when cancelled is false."
            n140 = for {
              shift-right: [w397] -> w378
              shift-left: w375 -> [w398]
              tunnel: w388 -> [w394] mode=indexing
              tunnel: w379 -> [w396]
              n141 = Empty String/Path?(string/path=w394) -> (empty?=w395:bool)
              n142 = case shown="False" w395 {
                tunnel: w398 -> [w402 w403]
                tunnel: [w401 w403] -> w397
                tunnel: w396 -> [w400 _]
                tunnel: w394 -> [w399 _]
                frame False {
                  # "Copies if path is not empty."
                  n143 = Copy(8:w402, 10:w400, 11:w399) -> (0:w401:errorcluster)  [unwired: 2 in, 2 out]
                }
                frame True {
                  # "Occurs if path is empty."
                }
              }
            }
            n144 = Unbundle By Name(w378) -> ("code"=w376:i32)
            n145 = case shown="10" w376 {
              selector: w376 -> [_ w391]
              tunnel: [w389 w392] -> w377
              tunnel: w378 -> [w389 w393]
              frame 0, Default {
              }
              frame 10 {
                n146 = call <vilib>:"Clear Errors.vi"("error in (no error)"=w393, "specific error code to clear (0: all)"=w391) -> ("error out"=w392:errorcluster)  [unwired: 4 in, 1 out]
                n147 = One Button Dialog(message="File already exists in the \nselected destination!!") -> ()  [unwired: 1 in, 1 out]
              }
            }
            n148 = Path To String(path=w379) -> (string=w386:string)
            n149 = Path To String(path=w387) -> (string=w385:string)
            n150 = Search and Replace String(input string=w386, search string=w385) -> (number of replacements=w384:i32)  [unwired: 6 in, 3 out]
            n151 = Greater Than 0?(x=w384) -> (x > 0?=w383:bool)
            n152 = case shown="True" w383 {
              tunnel: w377 -> [w407 w414]
              tunnel: [w407 w413] -> w382
              tunnel: w381 -> [w406 w410]
              tunnel: [w404 w408] -> w380
              tunnel: w379 -> [_ w409]
              frame False {
                n153 = Bundle By Name(cluster=w406, "SelectedFilePaths"=path[] []) -> (w404:T2)
              }
              frame True {
                n154 = Bundle By Name(cluster=w410, "NewSelectedPath"=w409) -> (w408:T2)
                n155 = call "QueueDriver.vi"("State"=T1 {"State"="RePopulateInExistFolder", "Data"=variant}, "error in (no error)"=w414, "Operations"=Operations."Enqueue") -> ("error out"=w413:errorcluster)  [unwired: 11 in, 1 out]
              }
            }
          }
          frame True {
            # "This case occurs when user cancels the dialog box."
            n156 = call <vilib>:"Clear Errors.vi"("error in (no error)"=w418) -> ("error out"=w417:errorcluster)  [unwired: 5 in, 1 out]
            n157 = One Button Dialog(message="User cancelled the copy operation!!!!") -> ()  [unwired: 1 in, 1 out]
          }
        }
      }
      frame "RePopulateInExistFolder" {
        # "Displays the copied folder in tree if its selected path is currently populated folder."
        n158 = Unbundle By Name(w420) -> ("NewSelectedPath"=w426:path, "FolderPathArray"=w427:path[], "SelectedFilePaths"=w425:path[])
        n159 = for {
          tunnel: w427 -> [w441] mode=indexing
          tunnel: w426 -> [w438]
          tunnel: [w439] -> w421
          tunnel: w425 -> [w440]
          shift-right: [w443] -> w424
          shift-left: w428 -> [w444]
          n160 = Equal?(x=w438, y=w441) -> (x = y?=w439:bool)
          n161 = Path To String(path=w438) -> (string=w442:string)
          n162 = case shown="True" w439 {
            tunnel: w444 -> [w445 w449]
            tunnel: [w445 w448] -> w443
            tunnel: w442 -> [_ w446]
            tunnel: w440 -> [_ w447]
            frame False {
            }
            frame True {
              n163 = for {
                tunnel: w446 -> [w455]
                shift-right: [w456] -> w448
                shift-left: w449 -> [w453]
                tunnel: w447 -> [w451] mode=indexing
                n164 = call "FileInformation.vi"("File Path"=w451, "error in (no error)"=w453) -> ("FileInfo"=w450:string[], "error out"=w452:errorcluster)  [unwired: 12 in]
                n165 = Strip Path(path=w451) -> (name=w454:string)  [unwired: 1 out]
                n166 = invoke on="Tree" class="Tree (strict)" method="Edit Tree Items.Add Item"(error in=w452, "Parent Tag"=w455, "Left Cell"=w454, "Child Text"=w450, "Child Tag"=w454) -> (error out=w456:errorcluster)  [unwired: 4 in, 8 out]
              }
            }
          }
        }
        n167 = case shown="False" w421 {
          tunnel: w424 -> [w433 w437]
          tunnel: [w430 w437] -> w423
          tunnel: w420 -> [w429 w436]
          tunnel: [w429 w435] -> w419
          frame False {
            n168 = call "QueueDriver.vi"("State"=T1 {"State"="RePopulateInNewFolder", "Data"=variant}, "error in (no error)"=w433, "Operations"=Operations."Enqueue") -> ("error out"=w430:errorcluster)  [unwired: 11 in, 1 out]
          }
          frame True {
            n169 = Bundle By Name(cluster=w436, "SelectedFilePaths"=path[] []) -> (w435:T2)
          }
        }
      }
      frame "RePopulateInNewFolder" {
        # "Populates the copied folder if its destination path is currently populated folder."
        n170 = Unbundle By Name(w460) -> ("NewSelectedPath"=w457:path, "FolderPathArray"=w467:path[], "SelectedFilePaths"=w462:path[])
        n171 = Strip Path(path=w457) -> (stripped path=w468:path)  [unwired: 1 out]
        n172 = for {
          tunnel: w468 -> [w478]
          tunnel: w467 -> [w485] mode=indexing
          shift-right: [w481] -> w465
          shift-left: w466 -> [w483]
          tunnel: [w479] -> w463
          tunnel: w457 -> [w477]
          stop <- w480 stop-if-true
          # "Populates the created new folder in tree"
          n173 = Path To String(path=w485) -> (string=w484:string)
          n174 = Path To String(path=w477) -> (string=w482:string)
          n175 = Equal?(x=w478, y=w485) -> (x = y?=w480:bool)
          n176 = Strip Path(path=w477) -> (name=w476:string)  [unwired: 1 out]
          n177 = case shown="True" w480 {
            tunnel: w484 -> [_ w491]
            tunnel: w483 -> [w487 w492]
            tunnel: w482 -> [w486 w488]
            tunnel: [w487 w490] -> w481
            tunnel: [w486 w488] -> w479
            tunnel: w476 -> [_ w489]
            frame False {
            }
            frame True {
              n178 = invoke on="Tree" class="Tree (strict)" method="Edit Tree Items.Add Item"(error in=w492, "Parent Tag"=w491, "Left Cell"=w489, "Child Tag"=w488) -> (error out=w490:errorcluster)  [unwired: 5 in, 8 out]
            }
          }
        }
        n179 = for {
          tunnel: w463 -> [w474]
          tunnel: w462 -> [w470] mode=indexing
          shift-right: [w475] -> w464
          shift-left: w465 -> [w472]
          # "Populates the copied files in tree"
          n180 = call "FileInformation.vi"("File Path"=w470, "error in (no error)"=w472) -> ("FileInfo"=w469:string[], "error out"=w471:errorcluster)  [unwired: 12 in]
          n181 = Strip Path(path=w470) -> (name=w473:string)  [unwired: 1 out]
          n182 = invoke on="Tree" class="Tree (strict)" method="Edit Tree Items.Add Item"(error in=w471, "Parent Tag"=w474, "Left Cell"=w473, "Child Text"=w469, "Child Tag"=w473) -> (error out=w475:errorcluster)  [unwired: 4 in, 8 out]
        }
        n183 = Bundle By Name(cluster=w460, "SelectedFilePaths"=path[] []) -> (w459:T2)
      }
      frame "Expand all" {
        # "This case expands/collapses all the nodes in the tree."
        n184 = Variant To Data(error in=w501, type=TRUE, Variant=w499) -> (data=w495:bool, error out=w497:errorcluster)
        n185 = Not(x=w495) -> (.not. x?=w494:bool)
        n186 = invoke on="Tree" class="Tree (strict)" method="Open/Close.Open/Close All"(error in=w497, "Open"=w494) -> (error out=w496:errorcluster)  [unwired: 2 in, 3 out]
      }
      frame "Column" {
        # "This case gets the the column number of selected item in tree."
        n187 = Variant To Data(error in=w509, type=0 ("Column"), Variant=w507) -> (data=w504:i32, error out=w508:errorcluster)
        n188 = Bundle By Name(cluster=w505, "Column"=w504) -> (w503:T2)
      }
      frame "/******** Front Panel Updates ********/" {
      }
      frame "FP Update" {
        # "This case updates the front panel indicators."
        n189 = Unbundle By Name(w515) -> ("Report"=→"Report":string)
      }
      frame "/********* Error Handling ********/" {
      }
      frame "Error" {
        # "This case handles the error if any occured."
        n190 = Unbundle By Name(w525) -> ("code"=w532:i32, "source"=w531:string)
        n191 = call <vilib>:"Clear Errors.vi"("error in (no error)"=w525) -> ("error out"=w534:errorcluster)  [unwired: 5 in, 1 out]
        n192 = Format Into String(format string="Error occurred in state \"%s\"!!\nError Code: %d\nError Source: %s\n\nDo you wish to continue?", error in=w534, w524, w532, w531) -> (resulting string=w530:string, error out=w527:errorcluster)  [unwired: 1 in]
        n193 = Unbundle By Name(w522) -> ("Stop user event"=w521:refnum<user-event>)
        n194 = Two Button Dialog(message=w530, 1:"Exit" ("F button name (\"Cancel\")"), 2:"Continue" ("T button name (\"OK\")")) -> (T button?=w526:bool)
        n195 = case shown="False" w526 {
          tunnel: w527 -> [w541 w542]
          tunnel: [w538 w542] -> w523
          tunnel: w521 -> [w535 _]
          frame False {
            # "This case occurs when user selects exit."
            n196 = Generate User Event(user event=w535, event data cluster=TRUE ("event data"), error in=w541) -> (error out=w539:errorcluster)  [unwired: 1 in, 1 out]
            n197 = call "QueueDriver.vi"("State"=T1 {"State"="Exit", "Data"=variant}, "error in (no error)"=w539, "Operations"=Operations."Enqueue") -> ("error out"=w538:errorcluster)  [unwired: 11 in, 1 out]
          }
          frame True {
            # "This case occurs when user selects to continue."
          }
        }
      }
      frame "/******** Stopping the running Vi ********/" {
      }
      frame "Exit" {
        # "This case stops the running vi."
        n198 = call "QueueDriver.vi"("error in (no error)"=w550, "Operations"=Operations."Flush") -> ("error out"=w551:errorcluster)  [unwired: 12 in, 1 out]
        n199 = call "QueueDriver.vi"("error in (no error)"=w551, "Operations"=Operations."Release") -> ("error out"=w549:errorcluster)  [unwired: 12 in, 1 out]
      }
    }
  }
  n200 = while {
    shift-right: [w555] -> w8
    shift-left: w19 -> [w556]
    tunnel: w18 -> [w557]
    tunnel: [w553] -> w9
    stop <- w554 stop-if-true
    n201 = event shown="[6] \"Copy Button\": Value Change" {
      selector: w557 -> [_ _ _ _ _ _ _ _]
      dyn-events: [_ _ _ _ _ _ _ _] -> w553
      timeout: 50 -> [_ _ _ _ _ _ _ _]
      tunnel: w556 -> [w559 w563 w576 w596 w607 w615 w619 w621]
      tunnel: [w559 w562 w575 w594 w606 w614 w618 w621] -> w555
      tunnel: [_ w564 _ _ _ _ _ TRUE] -> w554
      event Timeout {
        # "This event occurs when no other event occurs."
        n202 = event-data() -> ()  [unwired: 1 in, 1 out]
      }
      event Panel Close? {
        w564 = TRUE
        # "This event occurs when panel close is pressed and stops the running vi."
        n203 = event-data() -> ()  [unwired: 1 in, 1 out]
        n204 = call "QueueDriver.vi"("State"=T1 {"State"="Exit", "Data"=variant}, "error in (no error)"=w563, "Operations"=Operations."Enqueue") -> ("error out"=w562:errorcluster)  [unwired: 11 in, 1 out]
        n205 = event-data ("Event Filter Node")("Discard?"=w564) -> ()  [unwired: 1 in, 1 out]
      }
      event "FolderPath": Value Change {
        # "This event occurs when path value change is done by the user."
        n206 = event-data() -> ("NewVal"=w572:path)  [unwired: 1 in]
        n207 = To Variant(anything=w572) -> (Variant=w571:variant)
        n208 = Bundle By Name(cluster=T1 {"State"="", "Data"=variant} ("State"), "State"="ValidPath", "Data"=w571) -> (w566:T1)
        n209 = Bundle By Name(cluster=T1 {"State"="", "Data"=variant} ("State"), "State"="ClearTree") -> (w567:T1)
        n210 = Build Array(w567, w566) -> (w565:T1[])
        n211 = call "QueueDriver.vi"("State[]"=w565, "error in (no error)"=w576, "Operations"=Operations."Enqueue N") -> ("error out"=w575:errorcluster)  [unwired: 11 in, 1 out]
      }
      event "Tree": Mouse Down {
        # "This event occurs when a user selects an item in the tree."
        n212 = event-data() -> ("Coords"=w597:T4)  [unwired: 1 in]
        n213 = invoke on="Tree" class="Tree (strict)" method="Point To Row Column"(error in=w596, "Point"=w597) -> (error out=w595:errorcluster, "Tag"=w591:string, "Col"=w585:i32, "InGlyph"=w579:bool)  [unwired: 6 in, 4 out]
        n214 = To Variant(anything=w585) -> (Variant=w587:variant)
        n215 = To Variant(anything=w591) -> (Variant=w590:variant)
        n216 = To Variant(anything=w579) -> (Variant=w578:variant)
        n217 = Bundle By Name(cluster=T1 {"State"="", "Data"=variant} ("State"), "State"="Column", "Data"=w587) -> (w584:T1)
        n218 = Bundle By Name(cluster=T1 {"State"="", "Data"=variant} ("State"), "State"="GetTags", "Data"=w590) -> (w583:T1)
        n219 = Bundle By Name(cluster=T1 {"State"="", "Data"=variant} ("State"), "State"="CheckboxSelected", "Data"=w578) -> (w577:T1)
        n220 = Build Array(w584, w583, w577) -> (w582:T1[])
        n221 = call "QueueDriver.vi"("State[]"=w582, "error in (no error)"=w595, "Operations"=Operations."Enqueue N") -> ("error out"=w594:errorcluster)  [unwired: 11 in, 1 out]
      }
      event "SearchBar": Value Change {
        # "This event occurs when value change occurs in search bar."
        n222 = event-data() -> ("NewVal"=w604:string)  [unwired: 1 in]
        n223 = To Variant(anything=w604) -> (Variant=w602:variant)
        n224 = Bundle By Name(cluster=T1 {"State"="", "Data"=variant} ("State"), "State"="SearchTag", "Data"=w602) -> (w600:T1)
        n225 = Build Array(w600, T1 {"State"="SearchFolder", "Data"=variant} ("State")) -> (w598:T1[])
        n226 = call "QueueDriver.vi"("State[]"=w598, "error in (no error)"=w607, "Operations"=Operations."Enqueue N") -> ("error out"=w606:errorcluster)  [unwired: 11 in, 1 out]
      }
      event "Expand/Collapse": Value Change {
        # "This event occurs when Expand/Collapse button is pressed."
        n227 = event-data() -> ("NewVal"=w612:bool)  [unwired: 1 in]
        n228 = To Variant(anything=w612) -> (Variant=w610:variant)
        n229 = Bundle By Name(cluster=T1 {"State"="", "Data"=variant} ("State"), "State"="Expand all", "Data"=w610) -> (w608:T1)
        n230 = call "QueueDriver.vi"("State"=w608, "error in (no error)"=w615, "Operations"=Operations."Enqueue") -> ("error out"=w614:errorcluster)  [unwired: 11 in, 1 out]
      }
      event "Copy Button": Value Change {
        # "This event occurs when Copy button is pressed."
        n231 = event-data() -> ()  [unwired: 1 in, 1 out]
        n232 = call "QueueDriver.vi"("State"=T1 {"State"="CheckCopy", "Data"=variant}, "error in (no error)"=w619, "Operations"=Operations."Enqueue") -> ("error out"=w618:errorcluster)  [unwired: 11 in, 1 out]
      }
      event User Event {
        # "This user event stops the runing vi."
        n233 = event-data() -> ()  [unwired: 1 in, 1 out]
      }
    }
  }
  n234 = Unregister For Events(event registration refnum=w9, error in=w8) -> (error out=w7:errorcluster)
  n235 = Merge Errors(w7, w6) -> (w5:errorcluster)
  n236 = Destroy User Event(user event=w4, error in=w5) -> (error out=→"error out":errorcluster)
